vi "Auto_Drive (2).vi"(10 "Target":dbl format="%#_13g", 11 "Drive Effort":dbl=0.3) -> ()   [LabVIEW 2016]
uses:
  <vilib>/Rock Robotics/WPI/SafetyOutput/WPI_SafetyOutputConfigMenu.ctl
  Global 2.vi
panel:
  in  "Scaling Factor":dbl=16.0 format="%#_13g"
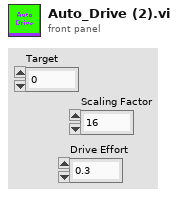
[diagram p1: front panel]
types:
  T1 = typedef "WPI_SafetyOutputConfigMenu.ctl" = enum16{"Enable", "Disable"}
  T2 = typedef "WPI_MotorControlDeviceRef.ctl" = cluster{"DeviceStatus":errorcluster, "Type":T3, "PWM":cluster{"PWM Channel":T4, "DeadBand":T5}, "CAN":cluster{"Device Number":u8, "SetOutput VI Ref":variant, "GetOutput VI Ref":variant, "Enable VI Ref":variant, "Disable VI Ref":variant, "Data":variant}, "Invert":bool}
  T3 = typedef "WPI_MotorControlType.ctl" = enum16{"PWM", "CAN"}
  T4 = typedef "FPGA_DIOPWMChannel.ctl" = enum8{"PWM 0", "PWM 1", "PWM 2", "PWM 3", "PWM 4", "PWM 5", "PWM 6", "PWM 7", "PWM 8", "PWM 9", "PWM MXP 0", "PWM MXP 1", "PWM MXP 2", "PWM MXP 3", "PWM MXP 4", "PWM MXP 5", "PWM MXP 6", "PWM MXP 7", "PWM MXP 8", "PWM MXP 9", "Invalid"}
  T5 = typedef "WPI_PWMDeadband.ctl" = cluster{"Name":string, "maxPositivePwm":i32, "minPositivePwm":i32, "centerPwm":i32, "maxNegativePwm":i32, "minNegativePwm":i32, "angularRange":u16}
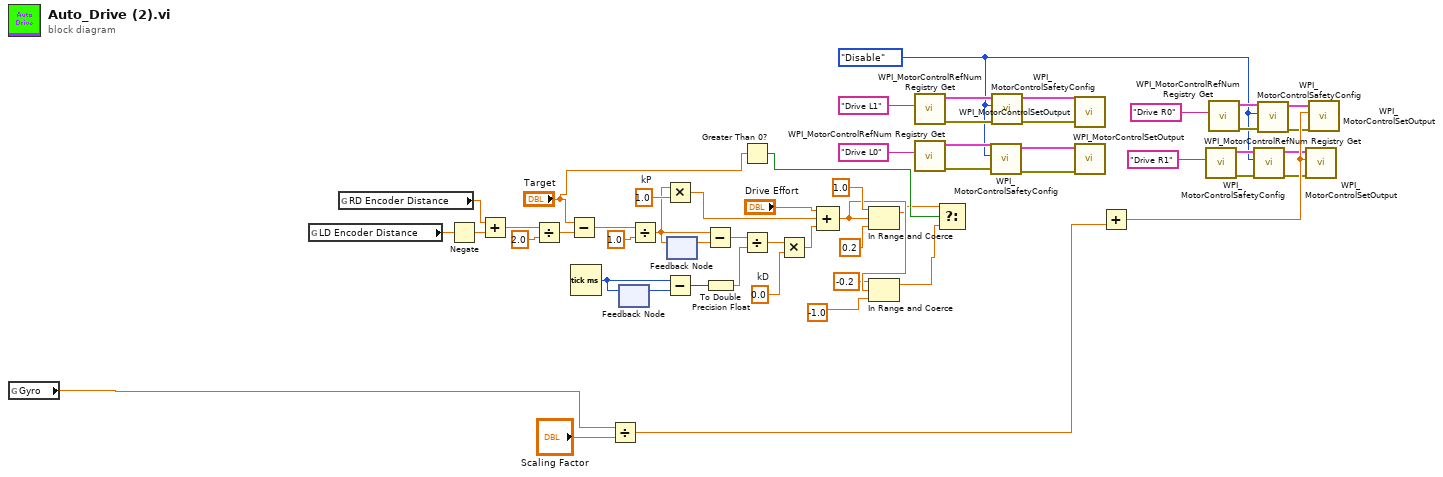
[diagram p0: block diagram]
diagram:
  w16 = 0.0  # kD
  w24 = 1.0  # kP
  w34 = WPI_SafetyOutputConfigMenu."Disable" ("mode")
  n1 = global read "Global 2.vi" "Gyro"() -> (w31:dbl)
  n2 = global read "Global 2.vi" "LD Encoder Distance"() -> (w30:dbl)
  n3 = global read "Global 2.vi" "RD Encoder Distance"() -> (w28:dbl)
  n4 = Negate(x=w30) -> (-x=w29:dbl)
  n5 = Add(x=w28, y=w29) -> (x+y=w27:dbl)
  n6 = Divide(x=w27, y=2.0) -> (x/y=w25:dbl)
  n7 = Subtract(x="Target", y=w25) -> (x-y=w10:dbl)
  n8 = Tick Count (ms)() -> (millisecond timer value=w21:u32)
  n9 = Divide(x=w31, y="Scaling Factor") -> (x/y=w32:dbl)
  n10 = feedback #1() -> (w22:u32)  [unwired: 1 in]
  n11 = feedback-in #1(w21) -> ()
  n12 = Divide(x=w10, y=1.0) -> (x/y=w8:dbl)
  n13 = Multiply(x=w8, y=w24) -> (x*y=w12:dbl)
  n14 = Subtract(x=w21, y=w22) -> (x-y=w19:u32)
  n15 = feedback-in #2(w8) -> ()
  n16 = feedback #2() -> (w23:dbl)  [unwired: 1 in]
  n17 = Subtract(x=w8, y=w23) -> (x-y=w20:dbl)
  n18 = To Double Precision Float(number=w19) -> (double precision float=w18:dbl)
  n19 = Greater Than 0?(x="Target") -> (x > 0?=w4:bool)
  n20 = Divide(x=w20, y=w18) -> (x/y=w17:dbl)
  n21 = Multiply(x=w17, y=w16) -> (x*y=w11:dbl)
  n22 = Compound Arithmetic op=ADD("Drive Effort", w12, w11) -> (w6:dbl)
  n23 = In Range and Coerce(upper limit=1.0, x=w6, lower limit=0.2) -> (coerced(x)=w3:dbl)  [unwired: 1 out]
  n24 = In Range and Coerce(upper limit=-0.2, x=w6, lower limit=-1.0) -> (coerced(x)=w2:dbl)  [unwired: 1 out]
  n25 = call <vilib>:"WPI_MotorControlRefNum Registry Get.vi"("refnum name"="Drive L1") -> ("error out"=w49:errorcluster, "MotorControlDevRef"=w50:T2)  [unwired: 9 in]
  n26 = call <vilib>:"WPI_MotorControlRefNum Registry Get.vi"("refnum name"="Drive L0") -> ("error out"=w45:errorcluster, "MotorControlDevRef"=w46:T2)  [unwired: 9 in]
  n27 = Select(t=w3, s=w4, f=w2) -> ()  [unwired: 1 out]
  n28 = call <vilib>:"WPI_MotorControlSafetyConfig.vi"("error in (no error)"=w45, "mode"=w34, "MotorControlDevRef"=w46) -> ("error out"=w43:errorcluster, "MotorControlDevRef"=w44:T2)  [unwired: 7 in]
  n29 = call <vilib>:"WPI_MotorControlSafetyConfig.vi"("error in (no error)"=w49, "mode"=w34, "MotorControlDevRef"=w50) -> ("error out"=w47:errorcluster, "MotorControlDevRef"=w48:T2)  [unwired: 7 in]
  n30 = call <vilib>:"WPI_MotorControlSetOutput.vi"("error in (no error)"=w47, "MotorControlDevRef"=w48) -> ()  [unwired: 7 in, 3 out]
  n31 = call <vilib>:"WPI_MotorControlSetOutput.vi"("error in (no error)"=w43, "MotorControlDevRef"=w44) -> ()  [unwired: 7 in, 3 out]
  n32 = Add(y=w32) -> (x+y=w51:dbl)  [unwired: 1 in]
  n33 = call <vilib>:"WPI_MotorControlRefNum Registry Get.vi"("refnum name"="Drive R1") -> ("error out"=w37:errorcluster, "MotorControlDevRef"=w38:T2)  [unwired: 9 in]
  n34 = call <vilib>:"WPI_MotorControlRefNum Registry Get.vi"("refnum name"="Drive R0") -> ("error out"=w41:errorcluster, "MotorControlDevRef"=w42:T2)  [unwired: 9 in]
  n35 = call <vilib>:"WPI_MotorControlSafetyConfig.vi"("error in (no error)"=w37, "mode"=w34, "MotorControlDevRef"=w38) -> ("error out"=w36:errorcluster, "MotorControlDevRef"=w35:T2)  [unwired: 7 in]
  n36 = call <vilib>:"WPI_MotorControlSafetyConfig.vi"("error in (no error)"=w41, "mode"=w34, "MotorControlDevRef"=w42) -> ("error out"=w40:errorcluster, "MotorControlDevRef"=w39:T2)  [unwired: 7 in]
  n37 = call <vilib>:"WPI_MotorControlSetOutput.vi"("error in (no error)"=w36, "Output"=w51, "MotorControlDevRef"=w35) -> ()  [unwired: 6 in, 3 out]
  n38 = call <vilib>:"WPI_MotorControlSetOutput.vi"("error in (no error)"=w40, "Output"=w51, "MotorControlDevRef"=w39) -> ()  [unwired: 6 in, 3 out]
